vi "Average Ai.vi"(0 "AIs":dbl[][](array[numeric])) -> (4 "Array":dbl[](array[numeric]))   [LabVIEW 2019]
uses:
  <userlib>/_MGI/1D Array/MGI Average/MGI Average (DBL[]).vi
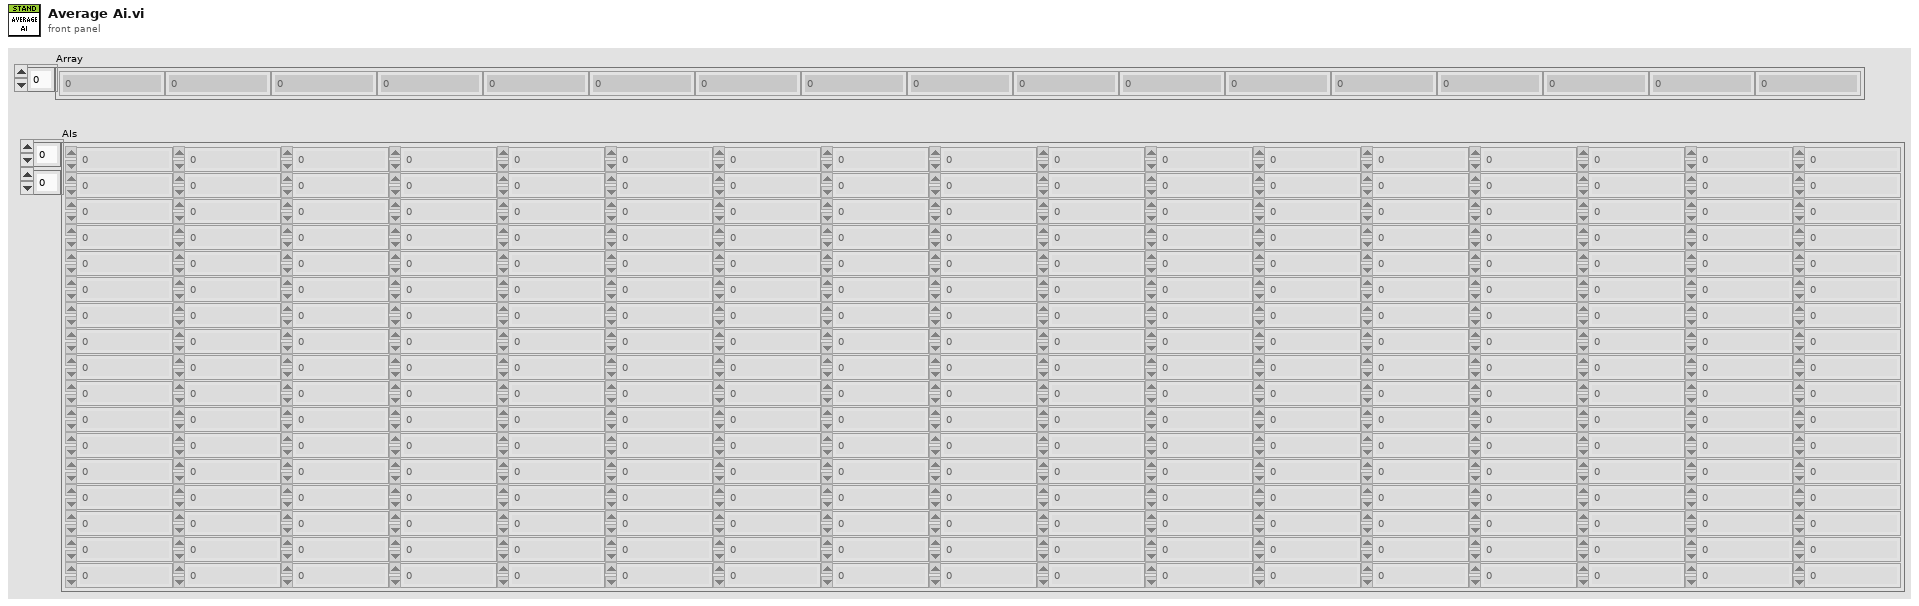
[diagram p1: front panel]
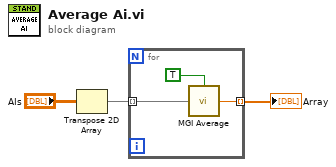
[diagram p0: block diagram]
diagram:
  n1 = Transpose 2D Array(2D array="AIs") -> (transposed array=w2:dbl[][])
  n2 = for {
    tunnel: w2 -> [w6] mode=indexing
    tunnel: [w4] -> w1 mode=indexing
    n3 = call-poly <userlib>:"MGI Average.vi"("Double[]"=w6, "Ignore NaN? (F)"=TRUE) -> ("Average"=w4:dbl)
  }
  "Array" <- w1
